vi "Command (write) - IH.vi"(7 "timeout ms (100)":i32=100, 8 "error in (no error)":errorcluster, 9 "Output":u8, 10 "IP":string, 11 "connection ID in":refnum<k16>) -> (0 "error out":errorcluster, 3 "connection ID out":refnum<k16>)   [LabVIEW 2016, in "SMD-7615.lvlib" / "eSCL.lvlib"]
doc: "IH - Immediate High Output\nSets an output high (open) immediately."
uses:
  eSCL.lvlib
  I32 Command and Param.ctl
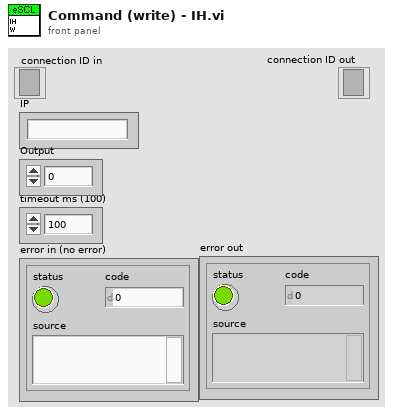
[diagram p1: front panel]
types:
  T1 = typedef "SMD-7615.lvlib/eSCL.lvlib/I32 Command and Param.ctl" = cluster{"Command":string, "I32 Parameler":i32, "I32 Parameler Default":i32, "I32 Parameler Coerece Upper":i32, "I32 Parameler Coerece Lower":i32}
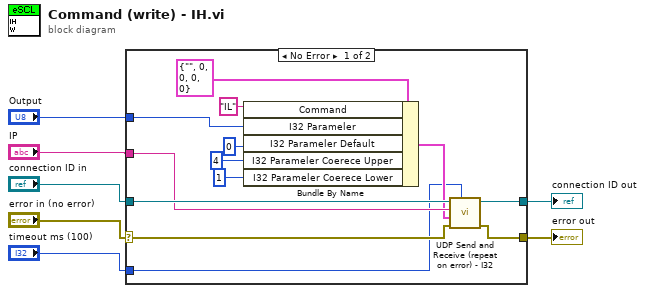
[diagram p0: block diagram]
diagram:
  n1 = case shown="No Error" "error in (no error)" {
    selector: "error in (no error)" -> [w12 w21]
    tunnel: "connection ID in" -> [w15 w22]
    tunnel: [w10 w22] -> w3
    tunnel: [w9 w21] -> w4
    tunnel: "IP" -> [w14 _]
    tunnel: "timeout ms (100)" -> [w11 _]
    tunnel: "Output" -> [w16 _]
    frame No Error {
      n2 = Bundle By Name(cluster=T1 {"Command"="", "I32 Parameler"=0, "I32 Parameler Default"=0, "I32 Parameler Coerece Upper"=0, "I32 Parameler Coerece Lower"=0} ("I32 Command & Param"), "Command"="IL", "I32 Parameler"=w16, "I32 Parameler Default"=0 ("DBL Parameler Default"), "I32 Parameler Coerece Upper"=4 ("DBL Parameler Coerece Upper"), "I32 Parameler Coerece Lower"=1 ("DBL Parameler Coerece Lower")) -> (w13:T1)
      n3 = call "UDP Send and Receive (repeat on error) - I32.vi"("timeout ms (100)"=w11, "error in (no error)"=w12, "I32 Command & Param"=w13, "IP"=w14, "connection ID in"=w15) -> ("error out"=w9:errorcluster, "connection ID out"=w10:refnum<k16>)  [unwired: 4 in, 1 out]
    }
    frame Error {
    }
  }
  "connection ID out" <- w3
  "error out" <- w4
